vi "CTRE_PigeonIMU_EnterCalibration.vi"(8 "error in (no error)":errorcluster, 10 "CalibrationMode":T1 items=["BootTareGryoAccel"=0, "Temperature"=1, "Magnetometer12Pt"=2, "Magnetometer360"=3, "Accelerometer"=5], 11 "PigeonIMUDevRef":T2={"DeviceStatus"={"status"=FALSE, "code"=0, "source"=""}, "Device Number"=0, "Type"=352321536, "Device ID"=0} {"Type" items=["CAN"=352321536, "TalonSRX"=33554432]}) -> (0 "error out":errorcluster, 3 "PigeonIMUDevRef":T2={"DeviceStatus"={"status"=FALSE, "code"=0, "source"=""}, "Device Number"=0, "Type"=352321536, "Device ID"=0} {"Type" items=["CAN"=352321536, "TalonSRX"=33554432]})   [LabVIEW 2016]
uses:
  <vilib>/Rock Robotics/WPI/ThirdParty/Sensors/Pigeon IMU/CTRE_PigeonIMU_DeviceRef.ctl
  <vilib>/Rock Robotics/WPI/ThirdParty/Sensors/Pigeon IMU/CTRE_PigeonIMU_ConnectionType.ctl
  <vilib>/Rock Robotics/WPI/ThirdParty/Sensors/Pigeon IMU/CTRE_PigeonIMU_CalibrationMode.ctl
  <vilib>/Rock Robotics/WPI/ThirdParty/Sensors/Pigeon IMU/CTRE_PigeonIMU_Params.ctl
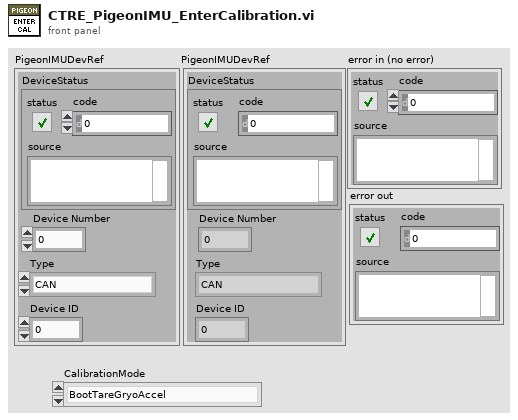
[diagram p1: front panel]
types:
  T1 = typedef "CTRE_PigeonIMU_CalibrationMode.ctl" = u16
  T2 = typedef "CTRE_PigeonIMU_DeviceRef.ctl" = cluster{"DeviceStatus":errorcluster, "Device Number":u8, "Type":T3, "Device ID":u32}
  T3 = typedef "CTRE_PigeonIMU_ConnectionType.ctl" = u32
  T4 = typedef "CTRE_PigeonIMU_Params.ctl" = u8
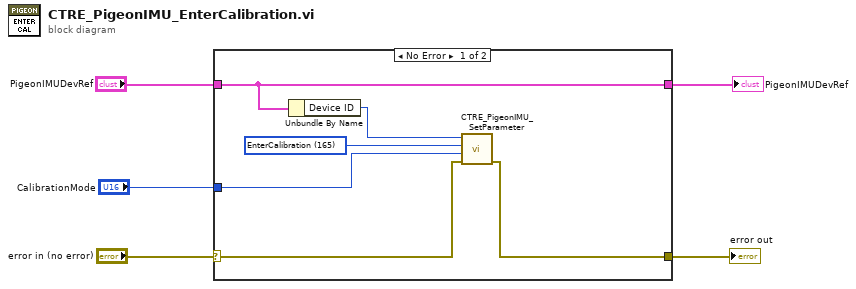
[diagram p0: block diagram]
diagram:
  n1 = case shown="No Error" "error in (no error)" {
    selector: "error in (no error)" -> [w8 w12]
    tunnel: [w7 w12] -> w4
    tunnel: [w11 w13] -> w2
    tunnel: "PigeonIMUDevRef" -> [w11 w13]
    tunnel: "CalibrationMode" -> [w6 _]
    frame No Error {
      w9 = T4 165 items=["YawOffset"=160, "CompassOffset"=161, "BetaGain"=162, "Reserved163"=163, "GyroNoMotionCal"=164, "EnterCalibration"=165, "FusedHeadingOffset"=166] ("Parameter")
      n2 = Unbundle By Name(w11) -> ("Device ID"=w10:u32)
      n3 = call <vilib>:"CTRE_PigeonIMU_SetParameter.vi"("error in (no error)"=w8, "Value"=w6, "Parameter"=w9, "Device ID (0)"=w10) -> ("error out"=w7:errorcluster)  [unwired: 6 in, 1 out]
    }
    frame Error {
    }
  }
  "PigeonIMUDevRef" <- w2
  "error out" <- w4
